vi "command engine process responses.vi"(8 "error out":errorcluster, 9 "State Variables":T1, 10 "Settings":T4 {"Compiled"."External Channels"."Channels" format="%.0x"; "Compiled"."External Channels"."Triggers" format="%.0x"}, 11 "Global Variables":T17) -> (0 "error out":errorcluster, 1 "State Variables out":T1, 2 "Settings out":T4 {"Compiled"."External Channels"."Channels" format="%.0x"; "Compiled"."External Channels"."Triggers" format="%.0x"}, 3 "Global Variables out":T17)   [LabVIEW 2018, in "Instrument Addon Engine.lvlib"]
uses:
  Instrument Addon Engine.lvlib
  Source/Addon/Support Libraries/Protections.lvlibp/Parent Protection/Protection.lvclass
  <vilib>/NI/Tools/Keyed Array/KeyedArray.ctl
  <vilib>/NI/Tools/Keyed Array/Tools_KeyedArray.lvlib
  <vilib>/NI/AMC/Message.ctl
  <vilib>/NI/AMC/AMC.lvlib
  <vilib>/NI/AMC/Message Queue.ctl
  Types/Engine State Variables.ctl
  Addon Shared/Types/Linked Channel Cluster.ctl
  Addon Shared/Instrument Addon Shared.lvlib
  Addon Shared/Types/Command Parameters.ctl
  <vilib>/NI VeriStand/Custom Device API/Data Reference.ctl
  <vilib>/NI VeriStand/Custom Device API/Custom Device API.lvlib
  Addon Shared/Types/Response Wait Type.ctl
  Addon Shared/Types/Response Parameters.ctl
  Addon Shared/Types/Response RT Configuration Cluster.ctl
  Addon Shared/Types/Message Generation Type.ctl
  Addon Shared/Types/Message Parameters.ctl
  Types/Commands RT Configuration Cluster.ctl
  Types/command engine global variables.ctl
  Addon Shared/Types/External Trigger Refs.ctl
  Addon Shared/Types/Compiled Settings.ctl
  Source/Addon/Support Libraries/Protocols.lvlibp/Protocol Parent/Protocol Parent.lvclass
  <vilib>/NI/NIVS Inline Async API/_VS Inline Async API/Process/Process.lvclass
  <vilib>/NI/NIVS Inline Async API/_Data Access Engine/Access Type Classes/ReadWrite/ReadWrite.lvclass
  <vilib>/NI/NI VeriStand Addon Network Comm/Engine/VeriStand Comm.lvclass
  <vilib>/NI/NIVS Inline Async API/_Data Access Engine/Access Type Classes/Write/Write.lvclass
  <vilib>/NI/NIVS Inline Async API/_Data Access Engine/Data Access Engine/Types/Write.DVR.ctl
  <vilib>/NI/NIVS Inline Async API/_Data Access Engine/Data Access Engine/Data Access Engine.lvclass
  <vilib>/NI/NIVS Inline Async API/_Data Access Engine/Access Type Classes/Read/Read.lvclass
  <vilib>/NI/NIVS Inline Async API/_Data Access Engine/Data Access Engine/Types/Read.DVR.ctl
  <vilib>/NI/NIVS Inline Async API/_Data Access Engine/Data Access Engine/Types/ReadWrite.DVR.ctl
  Addon Shared/Types/Command Channel Index.ctl
  Addon Shared/Types/Command Channel Indeces.ctl
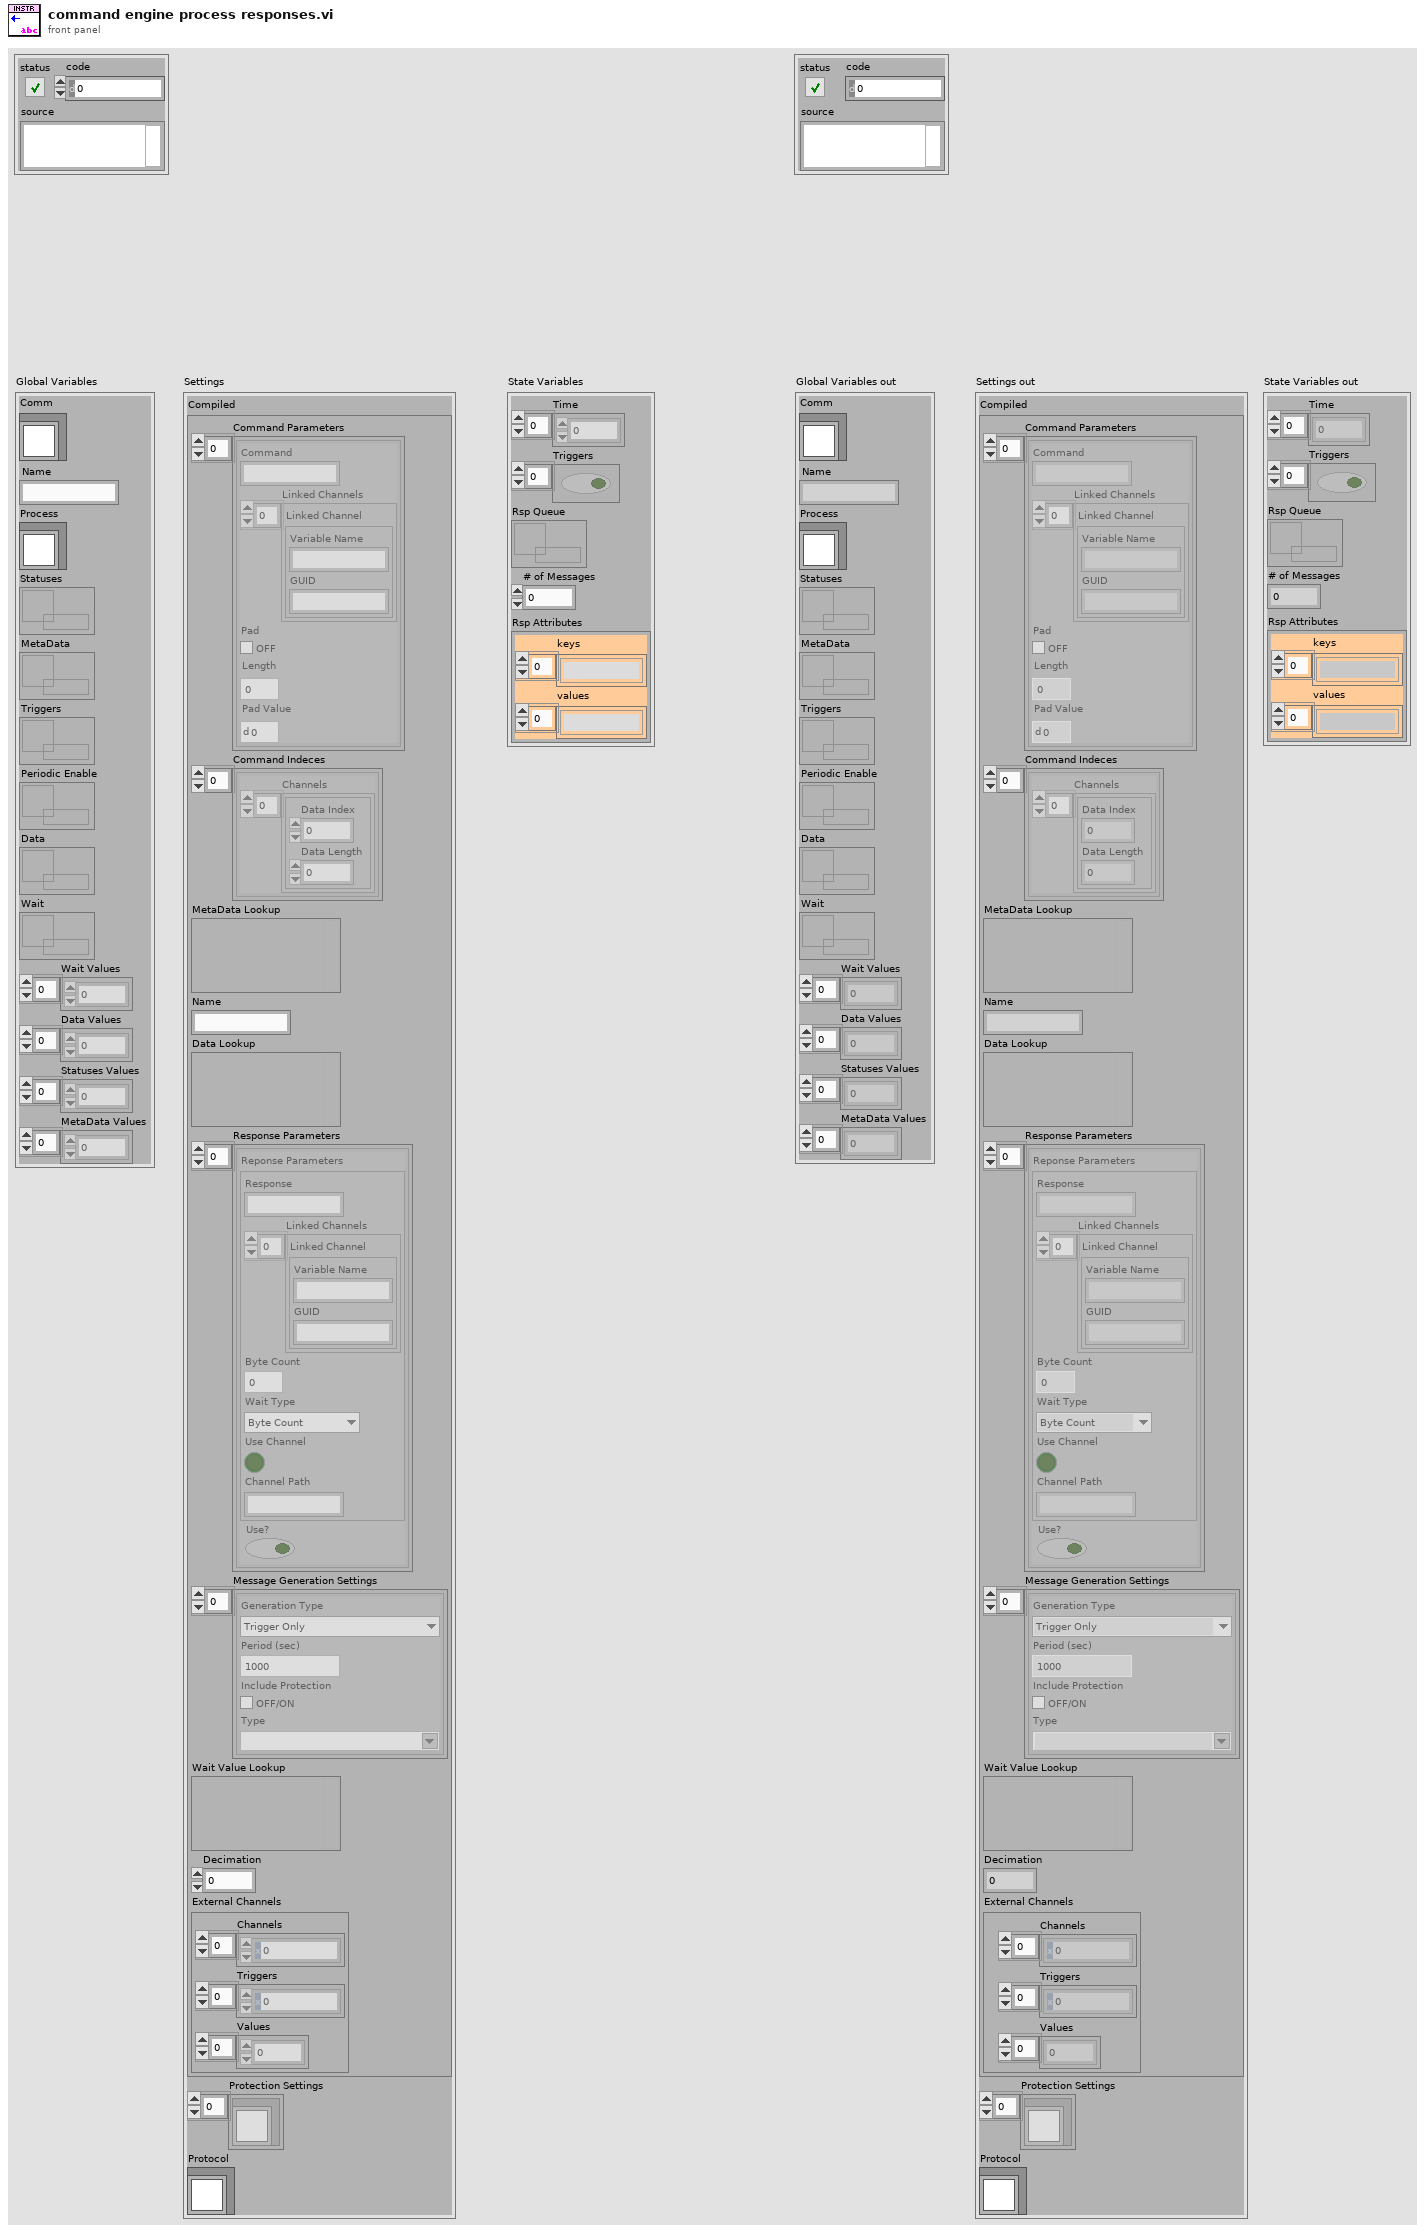
[diagram p1: front panel]
types:
  T1 = typedef "Instrument Addon Engine.lvlib/command engine global variables.ctl" = cluster{"Time":u32[], "Triggers":bool[], "Rsp Queue":T2, "# of Messages":i32, "Rsp Attributes":T3}
  T2 = typedef "AMC.lvlib/Message Queue.ctl" = refnum<queue>
  T3 = typedef "Tools_KeyedArray.lvlib/KeyedArray.ctl" = cluster{"keys":string[], "values":string[]}
  T4 = typedef "Instrument Addon Engine.lvlib/Commands RT Configuration Cluster.ctl" = cluster{"Compiled":T5, "Protection Settings":refnum<class "Protection.lvclass">[], "Protocol":refnum<class "Protocol Parent.lvclass">}
  T5 = typedef "Instrument Addon Shared.lvlib/Compiled Settings.ctl" = cluster{"Command Parameters":T6[], "Command Indeces":T8[], "MetaData Lookup":variant, "Name":string, "Data Lookup":variant, "Response Parameters":T10[], "Message Generation Settings":T13[], "Wait Value Lookup":variant, "Decimation":u32, "External Channels":T15}
  T6 = typedef "Instrument Addon Shared.lvlib/Command Parameters.ctl" = cluster{"Command":string, "Linked Channels":T7[], "Pad":bool, "Length":u32, "Pad Value":u8}
  T7 = typedef "Instrument Addon Shared.lvlib/Linked Channel Cluster.ctl" = cluster{"Variable Name":string, "GUID":string}
  T8 = typedef "Instrument Addon Shared.lvlib/Command Channel Indeces.ctl" = cluster{"Channels":T9[]}
  T9 = typedef "Instrument Addon Shared.lvlib/Command Channel Index.ctl" = cluster{"Data Index":i32, "Data Length":i32}
  T10 = typedef "Instrument Addon Shared.lvlib/Response RT Configuration Cluster.ctl" = cluster{"Reponse Parameters":T11, "Use?":bool}
  T11 = typedef "Instrument Addon Shared.lvlib/Response Parameters.ctl" = cluster{"Response":string, "Linked Channels":T7[], "Type Value":dbl, "Wait Type":T12, "Use Channel":bool, "Channel Path":string}
  T12 = typedef "Instrument Addon Shared.lvlib/Response Wait Type.ctl" = enum16{"Byte Count", "Wait sec"}
  T13 = typedef "Instrument Addon Shared.lvlib/Message Parameters.ctl" = cluster{"Generation Type":T14, "Period":dbl, "Include Protection":bool, "Type":string}
  T14 = typedef "Instrument Addon Shared.lvlib/Message Generation Type.ctl" = enum16{"Trigger Only", "Periodic & Trigger", "Value Change & Trigger"}
  T15 = typedef "Instrument Addon Shared.lvlib/External Trigger Refs.ctl" = cluster{"Channels":T16[], "Triggers":T16[], "Values":dbl[]}
  T16 = typedef "Custom Device API.lvlib/Data Reference.ctl" = i32
  T17 = typedef "Instrument Addon Engine.lvlib/Engine State Variables.ctl" = cluster{"Comm":refnum<class "VeriStand Comm.lvclass">, "Name":string, "Process":refnum<class "Process.lvclass">, "Statuses":T18, "MetaData":T19, "Triggers":T20, "Periodic Enable":T19, "Data":T18, "Wait":T19, "Wait Values":dbl[], "Data Values":dbl[], "Statuses Values":dbl[], "MetaData Values":dbl[]}
  T18 = typedef "Data Access Engine.lvlib/Data Access Engine.lvclass/Write.DVR.ctl" = refnum<data-value>
  T19 = typedef "Data Access Engine.lvlib/Data Access Engine.lvclass/Read.DVR.ctl" = refnum<data-value>
  T20 = typedef "Data Access Engine.lvlib/Data Access Engine.lvclass/ReadWrite.DVR.ctl" = refnum<data-value>
  T21 = typedef "Instrument Addon Shared.lvlib/Buffered RT Instrument Request.ctl" = cluster{"Response":string, "Error":errorcluster}
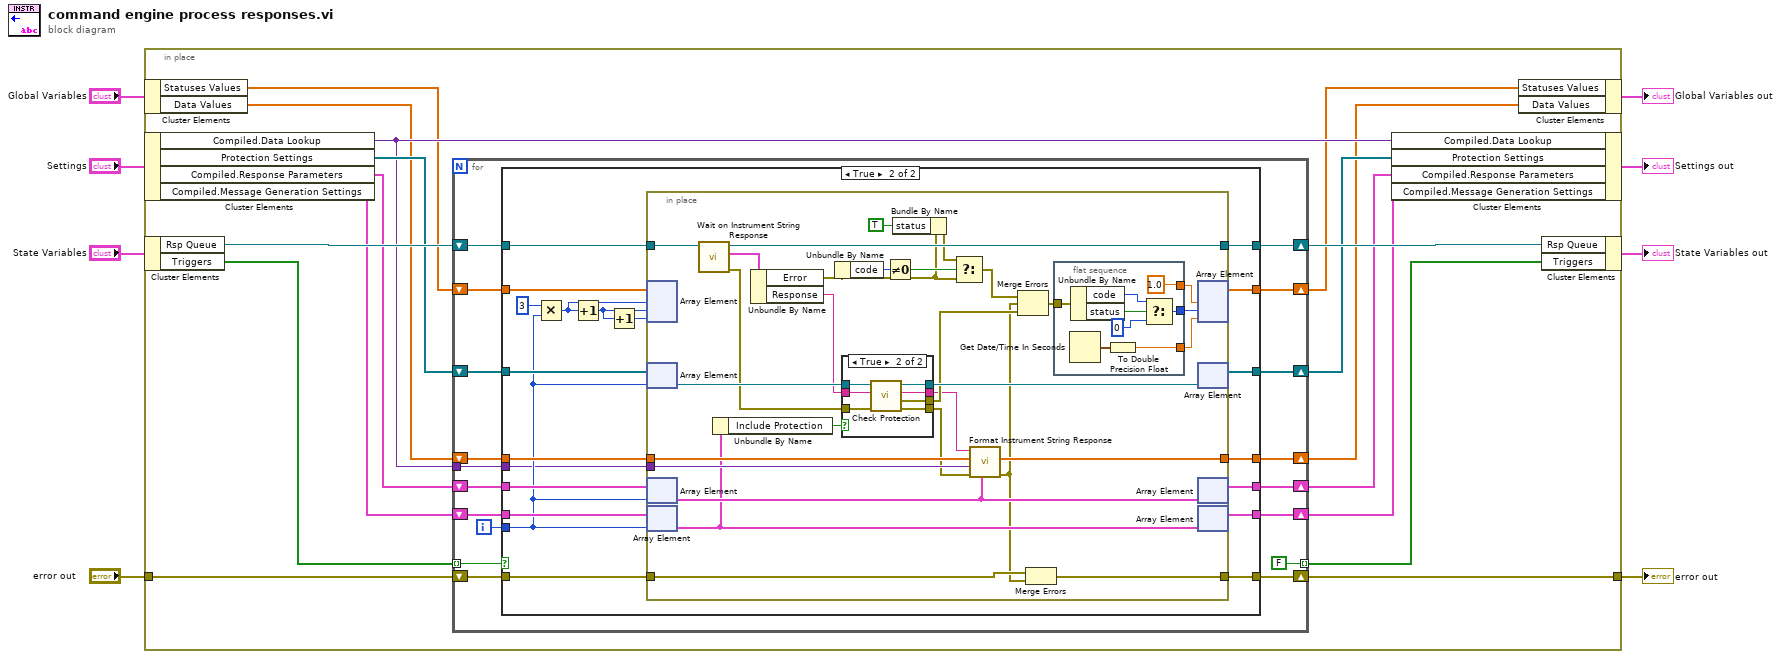
[diagram p0: block diagram]
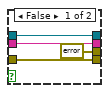
[diagram p3: hidden frame]
diagram:
  n1 = in-place {
    in-place-border: "error out" -> [w25]
    in-place-border: [w24] -> w8
    n2 = in-place-cluster #1("Global Variables") -> ("Statuses Values"=w10:dbl[], "Data Values"=w9:dbl[])
    n3 = in-place-cluster #2("Settings") -> ("Compiled.Data Lookup"=w13:variant, "Protection Settings"=w15:refnum<class "Protection.lvclass">[], "Compiled.Response Parameters"=w19:T10[], "Compiled.Message Generation Settings"=w18:T13[])
    n4 = in-place-cluster #3("State Variables") -> ("Rsp Queue"=w23:T2, "Triggers"=w22:bool[])
    n5 = for {
      shift-right: [w33] -> w11
      shift-left: w10 -> [w34]
      shift-right: [w43] -> w12
      shift-left: w9 -> [w41]
      shift-right: [w32] -> w14
      shift-left: w15 -> [w35]
      shift-right: [w28] -> w21
      shift-left: w23 -> [w29]
      shift-right: [w38] -> w16
      shift-left: w19 -> [w39]
      shift-right: [w36] -> w17
      shift-left: w18 -> [w37]
      tunnel: w13 -> [w30]
      shift-right: [w40] -> w24
      shift-left: w25 -> [w42]
      tunnel: w22 -> [w27] mode=indexing
      tunnel: [FALSE] -> w20 mode=indexing
      i -> [w31]
      n6 = case shown="True" w27 {
        tunnel: [w46 w70] -> w43
        tunnel: w42 -> [w47 w69]
        tunnel: w41 -> [w46 w68]
        tunnel: [w47 w67] -> w40
        tunnel: w39 -> [w45 w66]
        tunnel: [w45 w65] -> w38
        tunnel: w37 -> [w44 w64]
        tunnel: [w44 w63] -> w36
        tunnel: w35 -> [w50 w62]
        tunnel: w34 -> [w49 w61]
        tunnel: [w49 w58] -> w33
        tunnel: [w50 w57] -> w32
        tunnel: w31 -> [_ w56]
        tunnel: w30 -> [_ w55]
        tunnel: w29 -> [w48 w54]
        tunnel: [w48 w53] -> w28
        frame False {
        }
        frame True {
          n7 = Multiply(x=3, y=w56) -> (x*y=w59:i32)
          n8 = Increment(x=w59) -> (x+1=w51:i32)
          n9 = Increment(x=w51) -> (x+1=w52:i32)
          n10 = in-place {
            in-place-border: [w99] -> w70
            in-place-border: w69 -> [w98]
            in-place-border: w68 -> [w97]
            in-place-border: w55 -> [w96]
            in-place-border: [w95] -> w67
            in-place-border: w54 -> [w80]
            in-place-border: [w79] -> w53
            n11 = in-place-array #4(w61, w59, w51, w52) -> ()  [unwired: 3 out]
            n12 = in-place-array #5(w62, w56) -> (w92:refnum<class "Protection.lvclass">)
            n13 = in-place-array #6(w66, w56) -> (w94:T10)
            n14 = in-place-array #7(w64, w56) -> (w93:T13)
            n15 = call "Wait on Instrument String Response.vi"("Response Queue"=w80) -> ("error out"=w88:errorcluster, "Response"=w81:T21, "message queue out"=w79:T2)  [unwired: 8 in]
            n16 = Unbundle By Name(w93) -> ("Include Protection"=w85:bool)
            n17 = Unbundle By Name(w81) -> ("Error"=w75:errorcluster, "Response"=w84:string)
            n18 = Unbundle By Name(w75) -> ("code"=w78:i32)
            n19 = case shown="True" w85 {
              tunnel: w88 -> [w110 w118]
              tunnel: w84 -> [w111 w117]
              tunnel: [w111 w115] -> w83
              tunnel: [errorcluster {"status"=FALSE, "code"=0, "source"=""} ("error out") w113] -> w87
              tunnel: [w110 w114] -> w86
              tunnel: w92 -> [w108 w116]
              tunnel: [w108 w112] -> w90
              frame False {
              }
              frame True {
                n20 = call-dynamic "Check Protection.vi"("error in (no error)"=w118, "String in"=w117, "Protection in"=w116) -> ("error out"=w114:errorcluster, "Protection Error"=w113:errorcluster, "String out"=w115:string, "Protection out"=w112:refnum<class "Protection.lvclass">)  [unwired: 5 in]
              }
            }
            n21 = Not Equal To 0?(x=w78) -> (x != 0?=w77:bool)
            n22 = Bundle By Name(cluster=w75, "status"=TRUE) -> (w74:errorcluster)
            n23 = Select(t=w74, s=w77, f=w75) -> (s? t:f=w76:errorcluster)
            n24 = call "Format Instrument String Response.vi"("Response Parameters"=w94, "error in (no error)"=w86, "Data Lookup in"=w96, "Data"=w97, "Response"=w83) -> ("error out"=w82:errorcluster, "Data out"=w99:dbl[])  [unwired: 4 in, 1 out]
            n25 = Merge Errors(w76, w82, w87) -> (w89:errorcluster)
            n26 = Merge Errors(w98, w82) -> (w95:errorcluster)
            n27 = flat-sequence {
              tunnel: [1.0] -> w91
              tunnel: w89 -> [w106]
              tunnel: [w104] -> w72
              tunnel: [w100] -> w71
              frame #0 {
                n28 = Get Date/Time In Seconds() -> (seconds since 1Jan1904=w101:timestamp)
                n29 = Unbundle By Name(w106) -> ("code"=w103:i32, "status"=w105:bool)
                n30 = To Double Precision Float(number=w101) -> (double precision float=w100:dbl)
                n31 = Select(t=w103, s=w105, f=0) -> (s? t:f=w104:i32)
              }
            }
            n32 = in-place-array #4(w91, w72, w71) -> (w58:dbl[])  [unwired: 3 out]
            n33 = in-place-array #5(w90) -> (w57:refnum<class "Protection.lvclass">[])  [unwired: 1 out]
            n34 = in-place-array #6(w94) -> (w65:T10[])  [unwired: 1 out]
            n35 = in-place-array #7(w93) -> (w63:T13[])  [unwired: 1 out]
          }
        }
      }
    }
    n36 = in-place-cluster #2("Compiled.Data Lookup"=w13, "Protection Settings"=w14, "Compiled.Response Parameters"=w16, "Compiled.Message Generation Settings"=w17) -> (→"Settings out":T4)
    n37 = in-place-cluster #1("Statuses Values"=w11, "Data Values"=w12) -> (→"Global Variables out":T17)
    n38 = in-place-cluster #3("Rsp Queue"=w21, "Triggers"=w20) -> (→"State Variables out":T1)
  }
  "error out" <- w8
